vi "Write Max.vi"(8 "error in (no error)":errorcluster, 10 "Max":i32, 11 "LargeScrollbar in":refnum<class "LargeScrollbar.lvclass">) -> (0 "error out":errorcluster, 3 "LargeScrollbar out":refnum<class "LargeScrollbar.lvclass">)   [LabVIEW 2015, in "LargeScrollbar.lvclass"]
uses:
  LargeScrollbar.lvclass
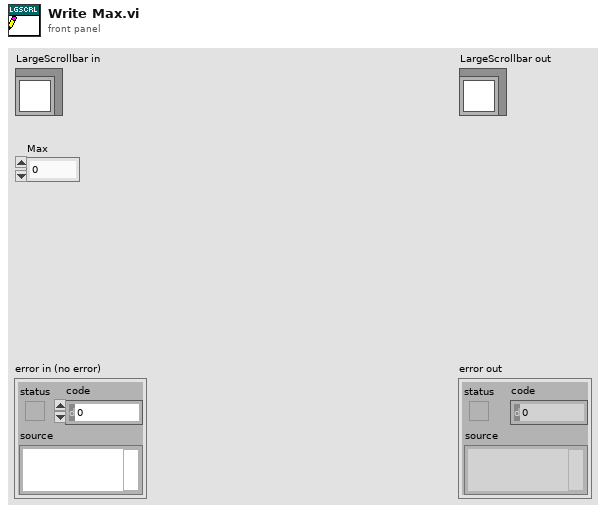
[diagram p1: front panel]
types:
  T1 = enum8{"Enabled", "Disabled", "Disabled and Grayed Out"}
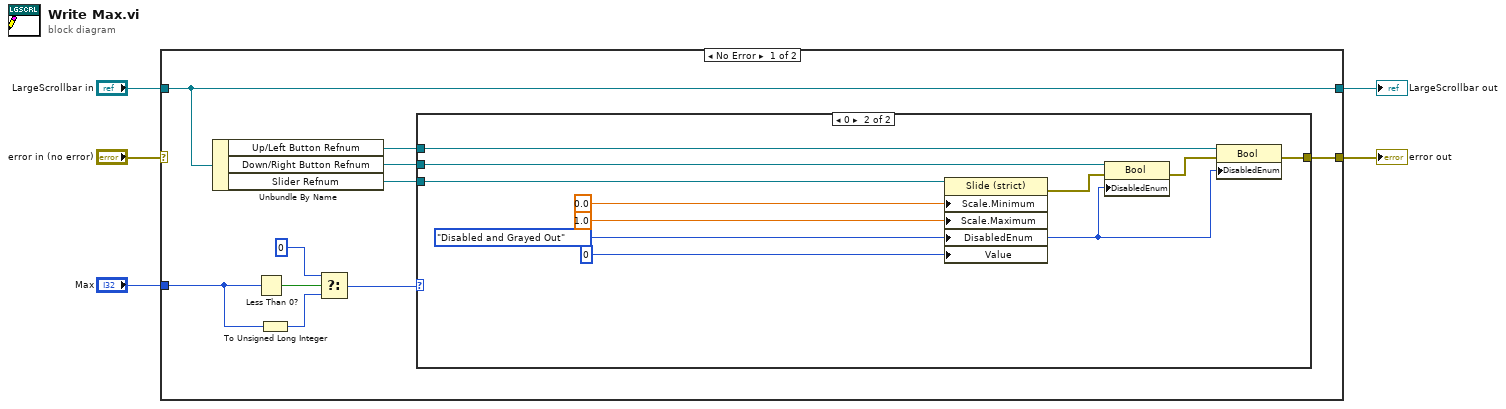
[diagram p0: block diagram]
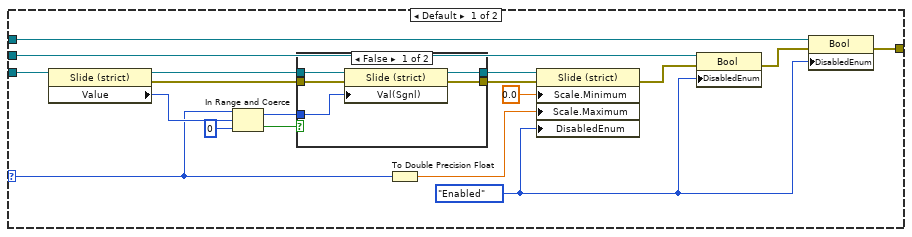
[diagram p2: hidden frame]
diagram:
  n1 = case shown="No Error" "error in (no error)" {
    selector: "error in (no error)" -> [_ w51]
    tunnel: [w11 w51] -> w4
    tunnel: [w15 w52] -> w2
    tunnel: "LargeScrollbar in" -> [w15 w52]
    tunnel: "Max" -> [w7 _]
    frame No Error {
      n2 = Unbundle By Name(w15) -> ("Up/Left Button Refnum"=w14:refnum<vi>, "Down/Right Button Refnum"=w13:refnum<vi>, "Slider Refnum"=w12:refnum<vi>)
      n3 = Less Than 0?(x=w7) -> (x < 0?=w10:bool)
      n4 = To Unsigned Long Integer(number=w7) -> (unsigned 32bit integer=w6:u32)
      n5 = Select(t=u32 0 ("Value"), s=w10, f=w6) -> (s? t:f=w9:u32)
      n6 = case shown="0" w9 {
        selector: w9 -> [w23 _]
        tunnel: w12 -> [w25 w50]
        tunnel: w13 -> [w30 w46]
        tunnel: w14 -> [w31 w45]
        tunnel: [w26 w41] -> w11
        frame Default {
          w29 = T1."Enabled" ("Disabled")
          n7 = property class="Slide (strict)"(reference=w25) -> (reference out=w21:refnum<vi>, error out=w19:errorcluster, "Value"=w24:u32)  [unwired: 1 in]
          n8 = In Range and Coerce(upper limit=w23, x=w24, lower limit=u32 0) -> (coerced(x)=w18:u32, In Range?=w20:bool)
          n9 = case shown="False" w20 {
            tunnel: w21 -> [w38 w40]
            tunnel: w19 -> [w37 w39]
            tunnel: w18 -> [w36 _]
            tunnel: [w35 w40] -> w17
            tunnel: [w34 w39] -> w16
            frame False {
              n10 = property class="Slide (strict)"(reference=w38, error in=w37, "Val(Sgnl)"=w36) -> (reference out=w35:refnum<vi>, error out=w34:errorcluster)
            }
            frame True {
            }
          }
          n11 = To Double Precision Float(number=w23) -> (double precision float=w33:dbl)
          n12 = property class="Slide (strict)"(reference=w17, error in=w16, "Scale.Minimum"=0.0 ("Scale.Range:Minimum"), "Scale.Maximum"=w33, "DisabledEnum"=w29) -> (error out=w28:errorcluster)  [unwired: 1 out]
          n13 = property class="Bool"(reference=w30, error in=w28, "DisabledEnum"=w29) -> (error out=w27:errorcluster)  [unwired: 1 out]
          n14 = property class="Bool"(reference=w31, error in=w27, "DisabledEnum"=w29) -> (error out=w26:errorcluster)  [unwired: 1 out]
        }
        frame 0 {
          w44 = T1."Disabled and Grayed Out" ("Disabled")
          n15 = property class="Slide (strict)"(reference=w50, "Scale.Minimum"=0.0 ("Scale.Range:Minimum"), "Scale.Maximum"=1.0 ("Scale.Range:Maximum"), "DisabledEnum"=w44, "Value"=u32 0) -> (error out=w43:errorcluster)  [unwired: 1 in, 1 out]
          n16 = property class="Bool"(reference=w46, error in=w43, "DisabledEnum"=w44) -> (error out=w42:errorcluster)  [unwired: 1 out]
          n17 = property class="Bool"(reference=w45, error in=w42, "DisabledEnum"=w44) -> (error out=w41:errorcluster)  [unwired: 1 out]
        }
      }
    }
    frame Error {
    }
  }
  "error out" <- w4
  "LargeScrollbar out" <- w2
